vi "Packet TX Only.vi"(2 "payload fifo":refnum<k21>, 3 "enable tx":bool=TRUE, 9 "udp payload length":u16, 13 "ready for input":T1) -> (6 "payload data":cluster{"Element":u8[], "Output Valid":bool}, 8 "start packet":bool, 10 "payload length":u16)   [LabVIEW 2017, in "My Network FPGA v1.lvlib"]
uses:
  My Network FPGA v1.lvlib
  <vilib>/rvi/DataTransferAndStorage/Container/Common/niFpgaContainerExecOnDevCompGetState.vi
  <vilib>/rvi/Emulation/niFpgaEmulationIsFPGAContextNoSignature.vi
  <vilib>/rvi/Emulation/niFpgaSctlEmulationGetInTimedLoop.vi
  <vilib>/rvi/errors/niFpgaSetErrorForExecOnDevCompSimple.vi
  <vilib>/rvi/eio/common/nirviEmuReportErrorAndStop.vi
  <vilib>/rvi/DataTransferAndStorage/Container/Common/niFpgaContainerGetUniqueNameForEmu.vi
  <vilib>/rvi/FIFO/Fifo_Resource/nirvififoEmulationSetSize.vi
  <vilib>/rvi/FIFO/Fifo_Resource/nirviFifoEmulationQueueMgr.vi
  <instcachedir>/0/nirviFifoEmulationQueueMgr_E5CAEC123FF24DC58D834DCA3CDAA9B5.lvgen/nirviFifoEmulationQueueMgr_E5CAEC123FF24DC58D834DCA3CDAA9B5_003.vi
  <vilib>/rvi/FIFO/Fifo_Resource/nirvififoEmulationDetermineInputValidOut.vi
  <vilib>/rvi/FIFO/Fifo_Resource/nirvififoEmulationCreateLock.vi
  <vilib>/rvi/Emulation/niFpgaProcessEmulError.vi
  <vilib>/rvi/FIFO/Fifo_Resource/nirvififoEmulationObtainLock.vi
  <vilib>/rvi/FIFO/Fifo_Resource/nirvififoEmulationReleaseLock.vi
  <vilib>/rvi/occurrence/nirviWaitOnOccurrenceBase.vi
  <vilib>/rvi/errors/nirviReportUnexpectedCaseInternalError.vi
  <vilib>/rvi/errors/nirviReportUnexpectedCaseInternalError (U32).vi
  <vilib>/Utility/error.llb/Clear Errors.vi
  <vilib>/rvi/interface/RandomDataEmulation/niFpgaRandomDataHandleErrors.vi
  <vilib>/rvi/DataTransferAndStorage/Container/XNode/niFpgaContainer.xnode
  <vilib>/rvi/FIFO/Fifo_Resource/niFpgaFifoEmulationRefIn.vi
  <instrlib>/_niInstr/Basic Elements/v1/FPGA/niInstr Basic Elements v1 FPGA.lvlib
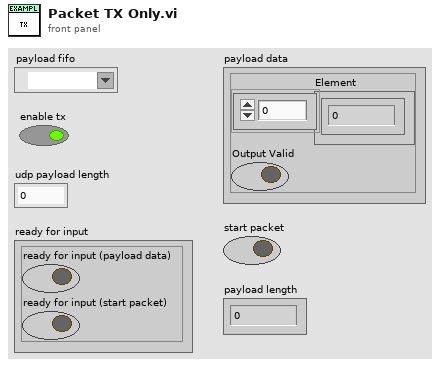
[diagram p1: front panel]
types:
  T1 = cluster{"ready for input (payload data)":bool, "ready for input (start packet)":bool}
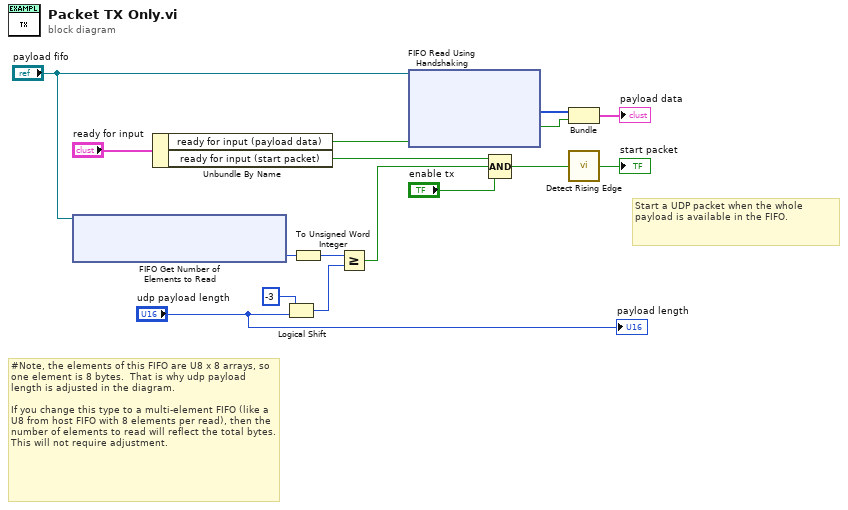
[diagram p0: block diagram]
diagram:
  # "#Note, the elements of this FIFO are U8 x 8 arrays, so one element is 8 bytes.  That is why udp payload length is adjusted in the diagram.\n\nIf you change this type to a multi-element FIFO (like a U8 from host FIFO with 8 elements per read), then the number of elements to read will reflect the total bytes.  This will not require adjustment."
  # "Start a UDP packet when the whole payload is available in the FIFO."
  n1 = xnode "FIFO Get Number of Elements to Read"("FIFO In"="payload fifo") -> ("Number of Elements to Read"=w8:u32)  [unwired: 1 out]
  n2 = Unbundle By Name("ready for input") -> ("ready for input (payload data)"=w4:bool, "ready for input (start packet)"=w10:bool)
  n3 = Logical Shift(y=i16 -3, x="udp payload length") -> (x << y=w14:u16)
  n4 = To Unsigned Word Integer(number=w8) -> (unsigned 16bit integer=w9:u16)
  n5 = Greater Or Equal?(x=w9, y=w14) -> (x >= y?=w11:bool)
  n6 = xnode "FIFO Read Using Handshaking"("Ready for Output"=w4, "FIFO In"="payload fifo") -> ("Element"=w5:u8[], "Output Valid"=w6:bool)  [unwired: 1 out]
  n7 = Compound Arithmetic op=AND(w10, w11, "enable tx") -> (w12:bool)
  n8 = Bundle("Element"=w5, "Output Valid"=w6) -> (→"payload data":cluster{"Element":u8[], "Output Valid":bool})  [unwired: 1 in]
  n9 = call <instrlib>:"Detect Rising Edge.vi"("signal"=w12) -> ("edge detected"=→"start packet":bool)  [unwired: 14 in]
  "payload length" <- "udp payload length"
